vi "ConvertBooleanToString.vi"(11 "True?":bool=TRUE) -> (3 "Boolean String":string)   [LabVIEW 2012, in "Keithley-7001.lvlib"]
uses:
  Keithley-7001.lvlib
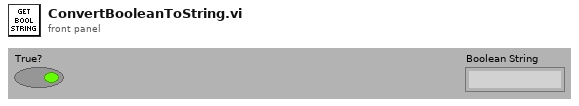
[diagram p1: front panel]
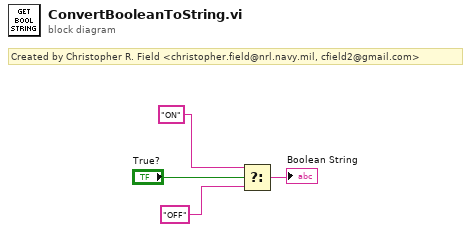
[diagram p0: block diagram]
diagram:
  # "Created by Christopher R. Field <christopher.field@nrl.navy.mil, cfield2@gmail.com>"
  n1 = Select(t="ON", s="True?", f="OFF") -> (s? t:f=→"Boolean String":string)
